vi "RTS Read TCP Command.vi"(7 "Client Side?":bool, 8 "error in (no error)":errorcluster, 11 "TCP Network Connection in":refnum<k5>) -> (0 "error out":errorcluster, 2 "TCP Command":string, 3 "TCP Network Connection out":refnum<k5>, 5 "Custom CMD?":bool)   [LabVIEW 2016]
uses:
  Type Definitions/RTS TCP Commands.ctl
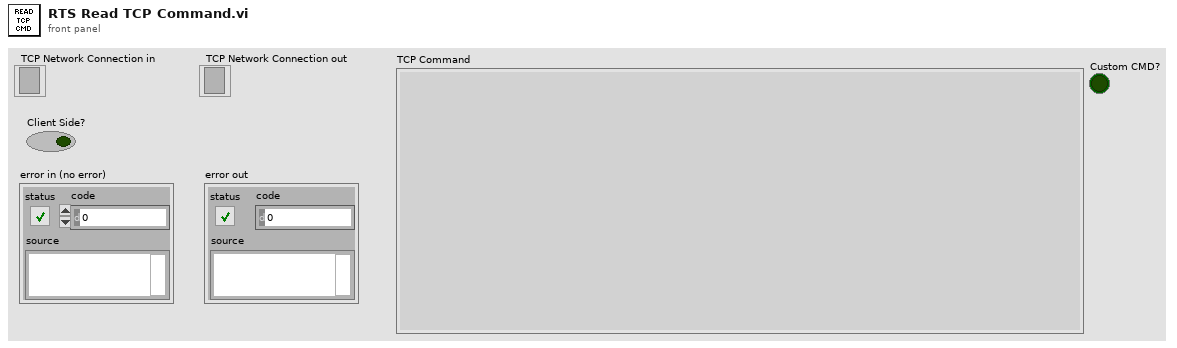
[diagram p1: front panel]
types:
  T1 = enum16{"Standard", "Buffered", "CRLF", "Immediate"}
  T2 = typedef "RTS TCP Commands.ctl" = string
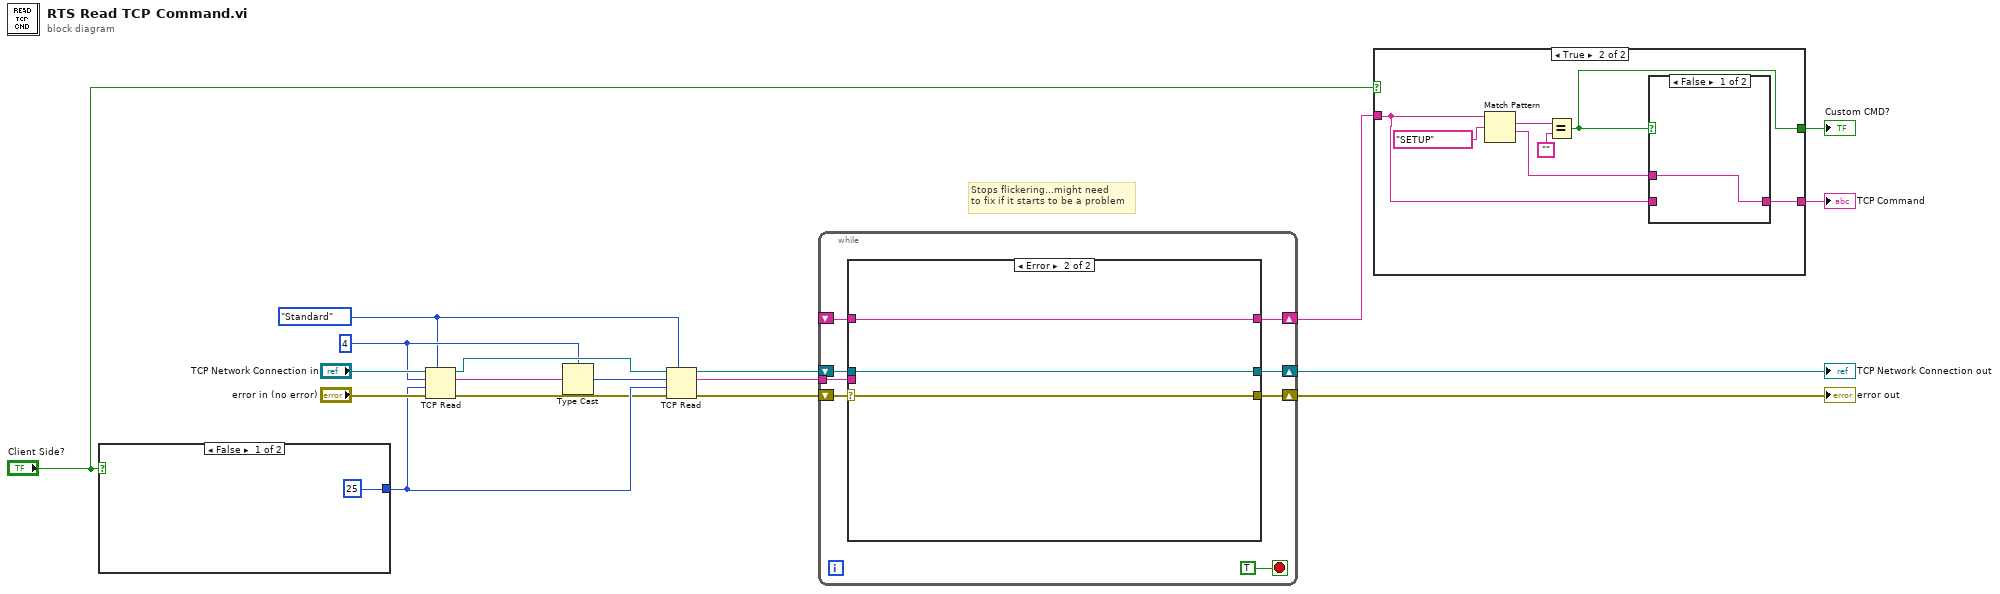
[diagram p0: block diagram]
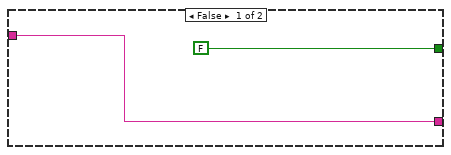
[diagram p2: hidden frame]
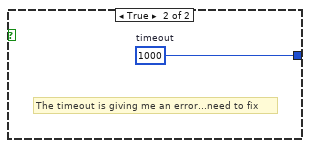
[diagram p5: hidden frame]
diagram:
  w5 = T1."Standard" ("mode (standard)")
  w13 = 4
  # "Stops flickering...might need\nto fix if it starts to be a problem"
  n1 = case shown="False" "Client Side?" {
    tunnel: [25 ("timeout") w20] -> w12
    frame False {
    }
    frame True {
      w20 = 1000  # timeout
      # "The timeout is giving me an error...need to fix"
    }
  }
  n2 = TCP Read(connection ID="TCP Network Connection in", bytes to read=w13, error in (no error)="error in (no error)", 7:w5, 9:w12) -> (connection ID out=w14:refnum<k5>, data out=w16:string, error out=w7:errorcluster)
  n3 = Type Cast(type=w13, x=w16) -> (*(type *) &x=w15:i32)
  n4 = TCP Read(connection ID=w14, bytes to read=w15, error in (no error)=w7, 7:w5, 9:w12) -> (connection ID out=w10:refnum<k5>, data out=w11:string, error out=w6:errorcluster)
  n5 = while {
    shift-right: [w23] -> w8
    shift-left: w6 -> [w28]
    shift-right: [w25] -> w9
    shift-left: w10 -> [w26]
    tunnel: w11 -> [w27]
    shift-right: [w24] -> w4
    shift-left: _ -> [w21]
    stop <- TRUE stop-if-true
    n6 = case shown="Error" w28 {
      selector: w28 -> [w29 w33]
      tunnel: w27 -> [w30 _]
      tunnel: w26 -> [w31 w32]
      tunnel: [w31 w32] -> w25
      tunnel: [w30 w34] -> w24
      tunnel: [w29 w33] -> w23
      tunnel: w21 -> [_ w34]
      frame No Error {
      }
      frame Error {
      }
    }
  }
  "error out" <- w8
  "TCP Network Connection out" <- w9
  n7 = case shown="True" "Client Side?" {
    tunnel: w4 -> [w35 w39]
    tunnel: [FALSE w40] -> w3
    tunnel: [w35 w38] -> w1
    frame False {
    }
    frame True {
      n8 = Match Pattern(string=w39, regular expression=T2 "SETUP" ("TCP Commands")) -> (match substring=w42:string, after substring=w37:string)  [unwired: 1 in, 2 out]
      n9 = Equal?(x=w42, y="") -> (x = y?=w40:bool)
      n10 = case shown="False" w40 {
        tunnel: w39 -> [_ w45]
        tunnel: [w44 w45] -> w38
        tunnel: w37 -> [w44 _]
        frame False {
        }
        frame True {
        }
      }
    }
  }
  "TCP Command" <- w1
  "Custom CMD?" <- w3
